vi "Q_data.vi"(7 "cmd":enum16{"create", "wirte", "read", "close"}(ring), 8 "error in":errorcluster, 10 "Strain_data":waveform(dbl)[](array[waveform]) caption="Res-Acc_data", 11 "Res-Acc_data":waveform(dbl)[](array[waveform])) -> (0 "error out":errorcluster, 3 "queue out":refnum<queue>)   [LabVIEW 2016]
uses:
  Ctrls/raw Q data.ctl
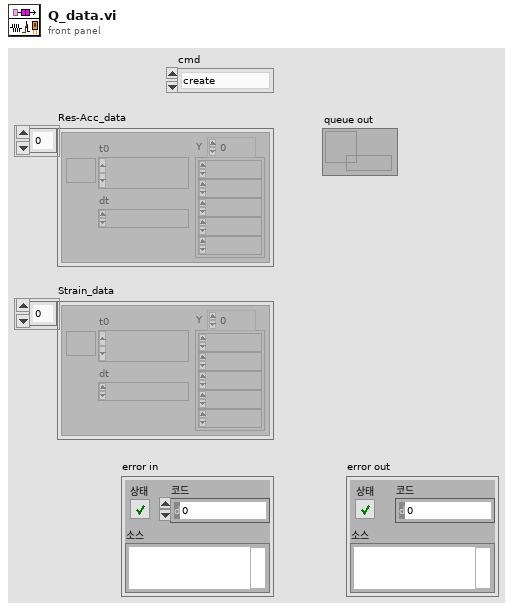
[diagram p1: front panel]
types:
  T1 = typedef "raw Q data.ctl" = cluster{"Res_data":waveform(dbl)[], "Acc_data":waveform(dbl), "Strain_data":waveform(dbl)[]}
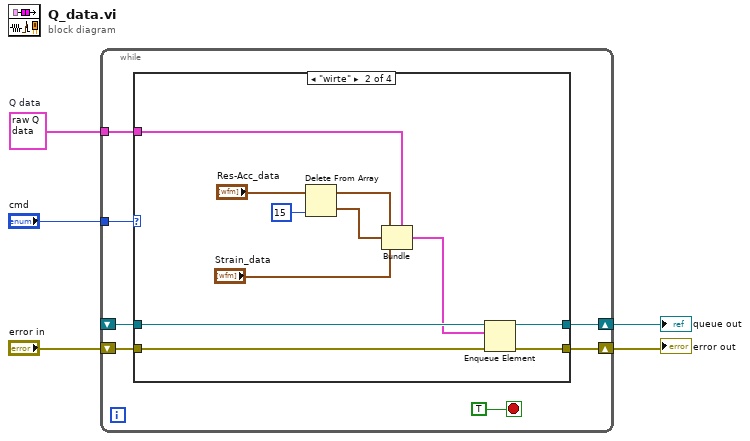
[diagram p0: block diagram]
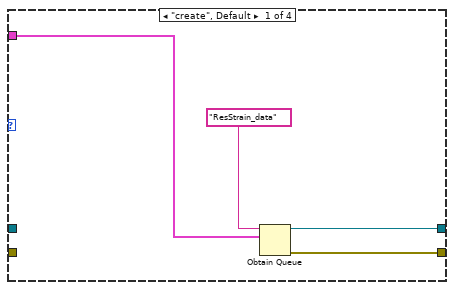
[diagram p2: hidden frame]
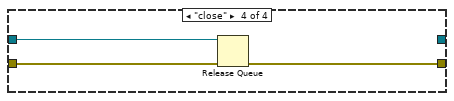
[diagram p4: hidden frame]
diagram:
  w1 = T1 {"Res_data"=[], "Acc_data"={"t0"=timestamp(0 s since 1904-01-01), "dt"=1.0, "Y"=[]}, "Strain_data"=[]}  # Q data
  n1 = while {
    tunnel: "cmd" -> [w11]
    shift-right: [w9] -> w3
    shift-left: "error in" -> [w10]
    shift-right: [w8] -> w2
    shift-left: _ -> [w7]
    tunnel: w1 -> [w6]
    stop <- TRUE stop-if-true
    n2 = case shown="\"wirte\"" w11 {
      tunnel: w10 -> [_ w27 w29 w32]
      tunnel: [w15 w26 w29 w31] -> w9
      tunnel: [w14 w25 w28 _] -> w8
      tunnel: w7 -> [_ w24 w28 w30]
      tunnel: w6 -> [w13 w17 _ _]
      frame "create", Default {
        n3 = Obtain Queue(name (unnamed)="ResStrain_data" ("이름(이름없음)"), element data type=w13) -> (queue out=w14:refnum<queue>, error out=w15:errorcluster)  [unwired: 3 in, 1 out]
      }
      frame "wirte" {
        n4 = Delete From Array(array="Res-Acc_data", index=15 ("인덱스 (행)")) -> (deleted portion=w18:waveform(dbl), array with subset deleted=w23:waveform(dbl)[])  [unwired: 1 in]
        n5 = Bundle(cluster=w17, "Res_data"=w23, "Acc_data"=w18, "Strain_data"="Strain_data") -> (w19:T1)
        n6 = Enqueue Element(queue=w24, element=w19, error in (no error)=w27) -> (queue out=w25:refnum<queue>, error out=w26:errorcluster)  [unwired: 1 in, 1 out]
      }
      frame "read" {
      }
      frame "close" {
        n7 = Release Queue(queue=w30, error in (no error)=w32) -> (error out=w31:errorcluster)  [unwired: 1 in, 2 out]
      }
    }
  }
  "error out" <- w3
  "queue out" <- w2
